vi "lab1.vi"() -> ()   [LabVIEW 2026]
panel:
  out "Output":string
  out "x <= y?":bool
  out "x >= y?":bool
  in  "Limit 2":dbl(knob) scale=80.0..100.0
  in  "Limit 1":dbl(knob) scale=75.0..90.0
  out "Numeric":dbl
  in  "stop":bool
  out "Waveform Chart":T1(graph)
  out "Thermometer":dbl(slide) scale=0.0..100.0
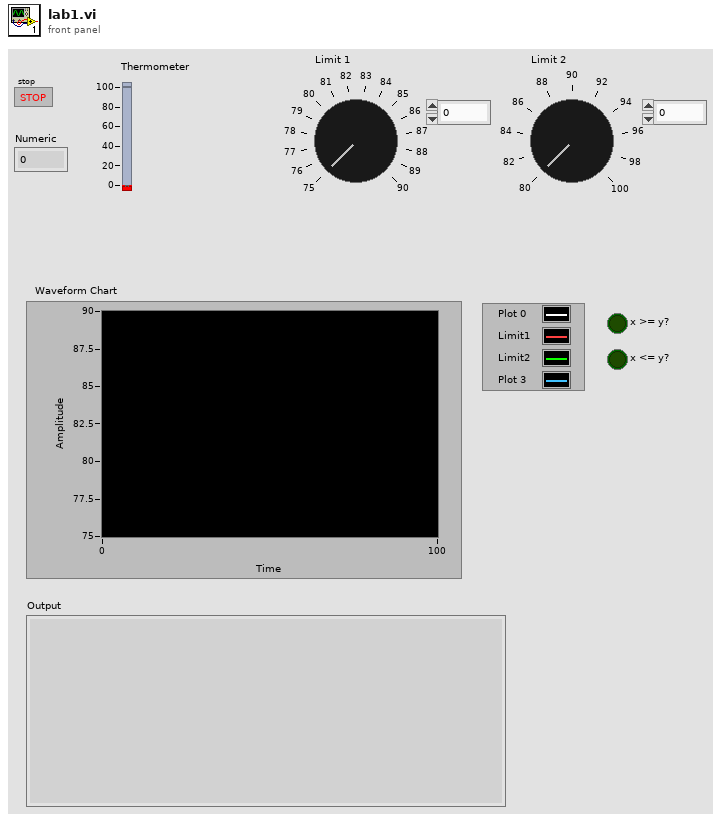
[diagram p1: front panel]
types:
  T1 = cluster{"temperature":dbl, "Limit 1":dbl, "Limit 2":dbl, dbl}
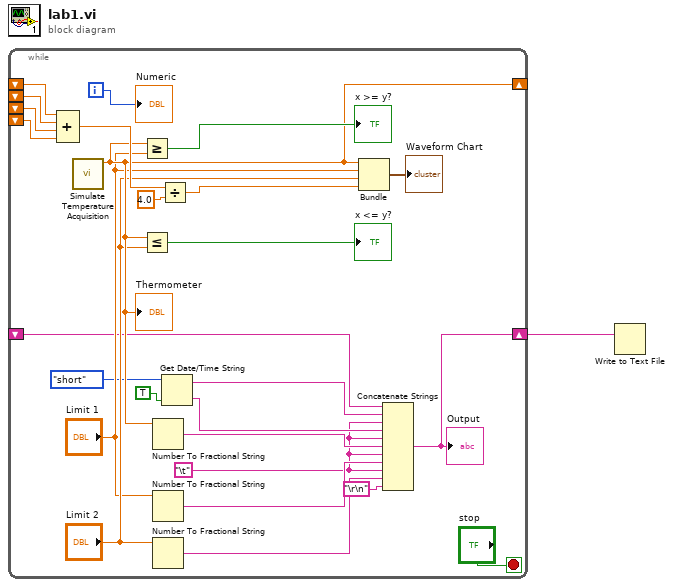
[diagram p0: block diagram]
diagram:
  n1 = while {
    shift-right: [w15] -> _
    shift-left: _ -> [w22]
    shift-left: _ -> [w21]
    shift-left: _ -> [w20]
    shift-left: _ -> [w19]
    shift-right: [w8] -> w1
    shift-left: _ -> [w5]
    i -> [w26]
    stop <- "stop" stop-if-true
    w2 = "\t"
    n2 = Compound Arithmetic op=ADD(w22, w21, w20, w19) -> (w18:dbl)
    n3 = call "Simulate Temperature Acquisition.vi"() -> ("temperature"=w15:dbl)  [unwired: 11 in]
    "Thermometer" <- w15
    n4 = Greater Or Equal?(x=w15, y="Limit 1") -> (x >= y?=→"x >= y?":bool)
    n5 = Less Or Equal?(x=w15, y="Limit 2") -> (x <= y?=→"x <= y?":bool)
    n6 = Number To Fractional String(number=w15) -> (F-format string=w14:string)  [unwired: 3 in]
    n7 = Number To Fractional String(number="Limit 1") -> (F-format string=w13:string)  [unwired: 3 in]
    n8 = Number To Fractional String(number="Limit 2") -> (F-format string=w10:string)  [unwired: 3 in]
    n9 = Divide(x=w18, y=4.0) -> (x/y=w16:dbl)
    n10 = Get Date/Time String(date format (0)=enum16{"short", "long", "abbreviated"}."short", want seconds? (F)=TRUE) -> (date string=w4:string, time string=w3:string)  [unwired: 1 in]
    n11 = Bundle("temperature"=w15, "Limit 1"="Limit 1", "Limit 2"="Limit 2", w16) -> (→"Waveform Chart":T1)  [unwired: 1 in]
    n12 = Concatenate Strings(w5, w4, w2, w3, w2, w14, w2, w13, w2, w10, "\r\n") -> (w8:string)
    "Output" <- w8
    "Numeric" <- w26
  }
  n13 = Write to Text File(text=w1) -> ()  [unwired: 3 in, 3 out]
